vi "test tree.vi"() -> ()   [LabVIEW 2014]
uses:
  spring action.ctl
panel:
  in  "Tree":string(tree)
  in  "indentation":u32[](array[numeric])=[0, 1, 1, 0]
  in  "symbols":u32[](array[numeric])=[0, 3, 2, 1]
  in  "bg colors":u32[](array[colorbox])=[16777164, 13434879, 13434828, 16777226]
  in  "fg colors":u32[](array[colorbox])=[0, 1442031, 16711680, 1985280]
  in  "item strings":string[][](array[string])=[["a", "1", ""], ["a1", "2", ""], ["a2", "3", ""], ["b", "4", ""]]
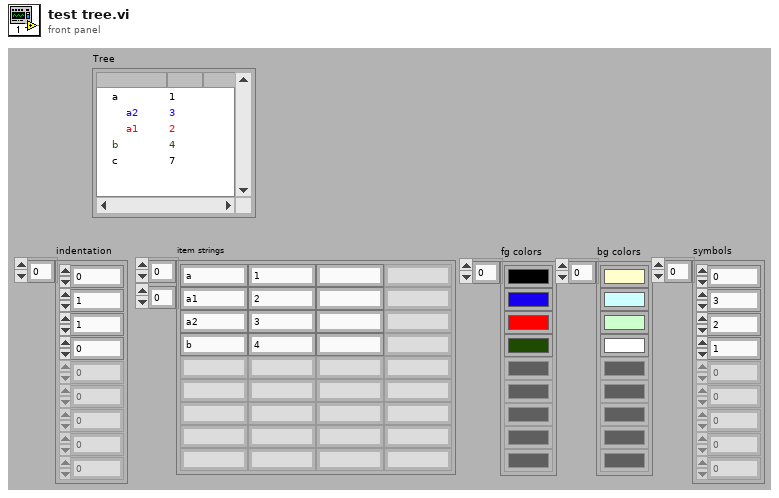
[diagram p1: front panel]
types:
  T1 = typedef "spring action.ctl" = enum16{"_init", "_add tree", "set itemstrings", "set fg colors", "set bg colors", "set symbols", "get tags", "get itemstrings", "get fg colors", "get bg colors", "get symbols", "empty tree", "update from tree", "find index of tag(s)", "set bold"}
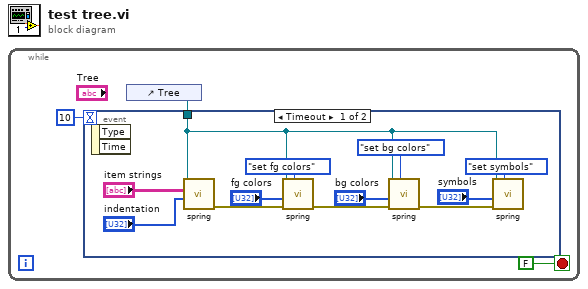
[diagram p0: block diagram]
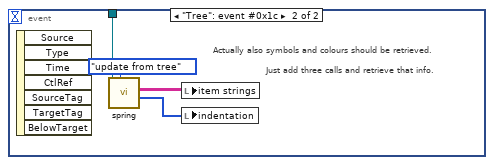
[diagram p2: hidden frame]
diagram:
  n1 = while {
    stop <- FALSE stop-if-true
    n2 = control-ref of="Tree"() -> (w1:refnum<vi>)
    n3 = event shown="[0] Timeout" {
      selector: _ -> [_ _]
      dyn-events: _ -> [_ _]
      timeout: 10 -> [_ _]
      tunnel: w1 -> [w8 w18]
      event Timeout {
        n4 = event-data() -> ()  [unwired: 1 in, 2 out]
        n5 = call "spring.vi"("indentation/item symbols/colors in"="indentation", "item strings in"="item strings", "tree ref"=w8) -> ("error out"=w11:errorcluster)  [unwired: 6 in, 2 out]
        n6 = call "spring.vi"("action (set itemstrings)"=spring_action."set fg colors" ("action (set)"), "error in (no error)"=w11, "indentation/item symbols/colors in"="fg colors", "tree ref"=w8) -> ("error out"=w10:errorcluster)  [unwired: 5 in, 2 out]
        n7 = call "spring.vi"("action (set itemstrings)"=spring_action."set bg colors" ("action (set)"), "error in (no error)"=w10, "indentation/item symbols/colors in"="bg colors", "tree ref"=w8) -> ("error out"=w9:errorcluster)  [unwired: 5 in, 2 out]
        n8 = call "spring.vi"("action (set itemstrings)"=spring_action."set symbols" ("action (set)"), "error in (no error)"=w9, "indentation/item symbols/colors in"="symbols", "tree ref"=w8) -> ()  [unwired: 5 in, 3 out]
      }
      event "Tree": event #0x1c {
        # "Just add three calls and retrieve that info."
        # "Actually also symbols and colours should be retrieved."
        n9 = event-data() -> ()  [unwired: 1 in, 7 out]
        n10 = call "spring.vi"("action (set itemstrings)"=spring_action."update from tree" ("action (set)"), "tree ref"=w18) -> ("item symbols/colors out"=w16:u32[], "item strings out"=w19:string[][])  [unwired: 7 in, 1 out]
        n11 = local write "item strings"(w19) -> ()
        n12 = local write "indentation"(w16) -> ()
      }
    }
  }
